vi "test-trajectory-generator-get.vi"(11 "traj_config":T4 {"End Velocity" format="%20.4f"; "StartVelocity" format="%20.4f"; "Max Acceleration" format="%20.4f"; "MaxVelocity" format="%20.4f"}) -> (0 "error out":errorcluster, 3 "TRAJECTORY":T5 {"States"."POSE"."ROTATION"."SIN" format="%13.4f"; "States"."POSE"."ROTATION"."COS" format="%13.4f"; "States"."POSE"."ROTATION"."VALUE" format="%13.4f"; "States"."POSE"."TRANSLATION"."Y" format="%14.3f"; "States"."POSE"."TRANSLATION"."X" format="%14.3f"; "TotalTImeSecs" format="%20.3f"}, 4 "Waypoints":T1[](array[typedef]) {"ROTATION"."SIN" format="%13.4f"; "ROTATION"."COS" format="%13.4f"; "ROTATION"."VALUE" format="%13.4f"; "TRANSLATION"."Y" format="%14.3f"; "TRANSLATION"."X" format="%14.3f"})   [LabVIEW 2019]
uses:
  <vilib>/Rock Robotics/WPI/ThirdParty/JAS_Junk/TrajLib/TRAJECTORY.ctl
  <vilib>/Rock Robotics/WPI/ThirdParty/JAS_Junk/TrajLib/TRAJ_STATE.ctl
  <vilib>/Rock Robotics/WPI/ThirdParty/JAS_Junk/TrajLib/POSE2D.ctl
  <vilib>/Rock Robotics/WPI/ThirdParty/JAS_Junk/TrajLib/TRANSLATION2D.ctl
  <vilib>/Rock Robotics/WPI/ThirdParty/JAS_Junk/TrajLib/ROTATION2D.ctl
  <vilib>/Rock Robotics/WPI/ThirdParty/JAS_Junk/TrajLib/TRAJ_CONFIG.ctl
  <vilib>/Rock Robotics/WPI/ThirdParty/JAS_Junk/TrajLib/DISPLAY_WAYPOINT.ctl
  <vilib>/Rock Robotics/WPI/ThirdParty/JAS_Junk/TrajLib/Rotation2d_CreateAngle.vi
  <vilib>/Rock Robotics/WPI/ThirdParty/JAS_Junk/TrajLib/Pose2d_TransformBy.vi
  <vilib>/Rock Robotics/WPI/ThirdParty/JAS_Junk/TrajLib/Translation2d_RotateBy.vi
  <vilib>/Rock Robotics/WPI/ThirdParty/JAS_Junk/TrajLib/Translation2d_Plus.vi
  <vilib>/Rock Robotics/WPI/ThirdParty/JAS_Junk/TrajLib/Rotation2d_Plus.vi
  <vilib>/Rock Robotics/WPI/ThirdParty/JAS_Junk/TrajLib/Pose2d_New_TRRO.vi
  <vilib>/Rock Robotics/WPI/ThirdParty/JAS_Junk/TrajLib/Rotation2d_RotateBy.vi
  <vilib>/Rock Robotics/WPI/ThirdParty/JAS_Junk/TrajLib/Rotation2d_CreateXY.vi
  <vilib>/Rock Robotics/WPI/ThirdParty/JAS_Junk/TrajLib/Util_CalcDist.vi
  <vilib>/Rock Robotics/WPI/ThirdParty/JAS_Junk/TrajLib/Trajectory_Library.lvlib
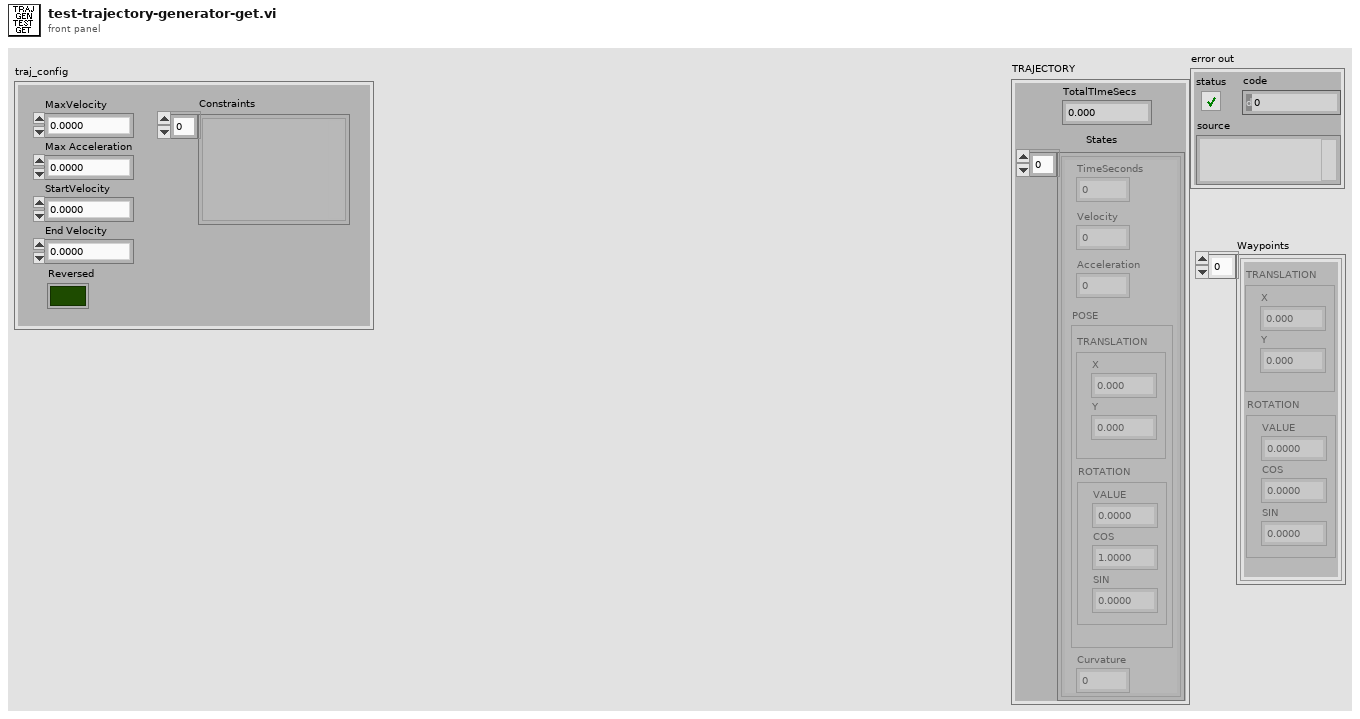
[diagram p1: front panel]
types:
  T1 = typedef "Trajectory_Library.lvlib/POSE2D.ctl" = cluster{"TRANSLATION":T2, "ROTATION":T3}
  T2 = typedef "Trajectory_Library.lvlib/TRANSLATION2D.ctl" = cluster{"X":dbl, "Y":dbl}
  T3 = typedef "Trajectory_Library.lvlib/ROTATION2D.ctl" = cluster{"VALUE":dbl, "COS":dbl, "SIN":dbl}
  T4 = typedef "Trajectory_Library.lvlib/TRAJ_CONFIG.ctl" = cluster{"MaxVelocity":dbl, "Max Acceleration":dbl, "StartVelocity":dbl, "End Velocity":dbl, "Reversed":bool, "Constraints":variant[]}
  T5 = typedef "Trajectory_Library.lvlib/TRAJECTORY.ctl" = cluster{"TotalTImeSecs":dbl, "States":T6[]}
  T6 = typedef "Trajectory_Library.lvlib/TRAJ_STATE.ctl" = cluster{"TimeSeconds":dbl, "Velocity":dbl, "Acceleration":dbl, "POSE":T1, "Curvature":dbl}
  T7 = typedef "Trajectory_Library.lvlib/TRANSFORM2D.ctl" = cluster{"TRANSLATION":T2, "ROTATION":T3, "xF":bool}
  T8 = typedef "Trajectory_Library.lvlib/DISPLAY_WAYPOINT.ctl" = cluster{"X":dbl, "Y":dbl, "ANGLE":dbl}
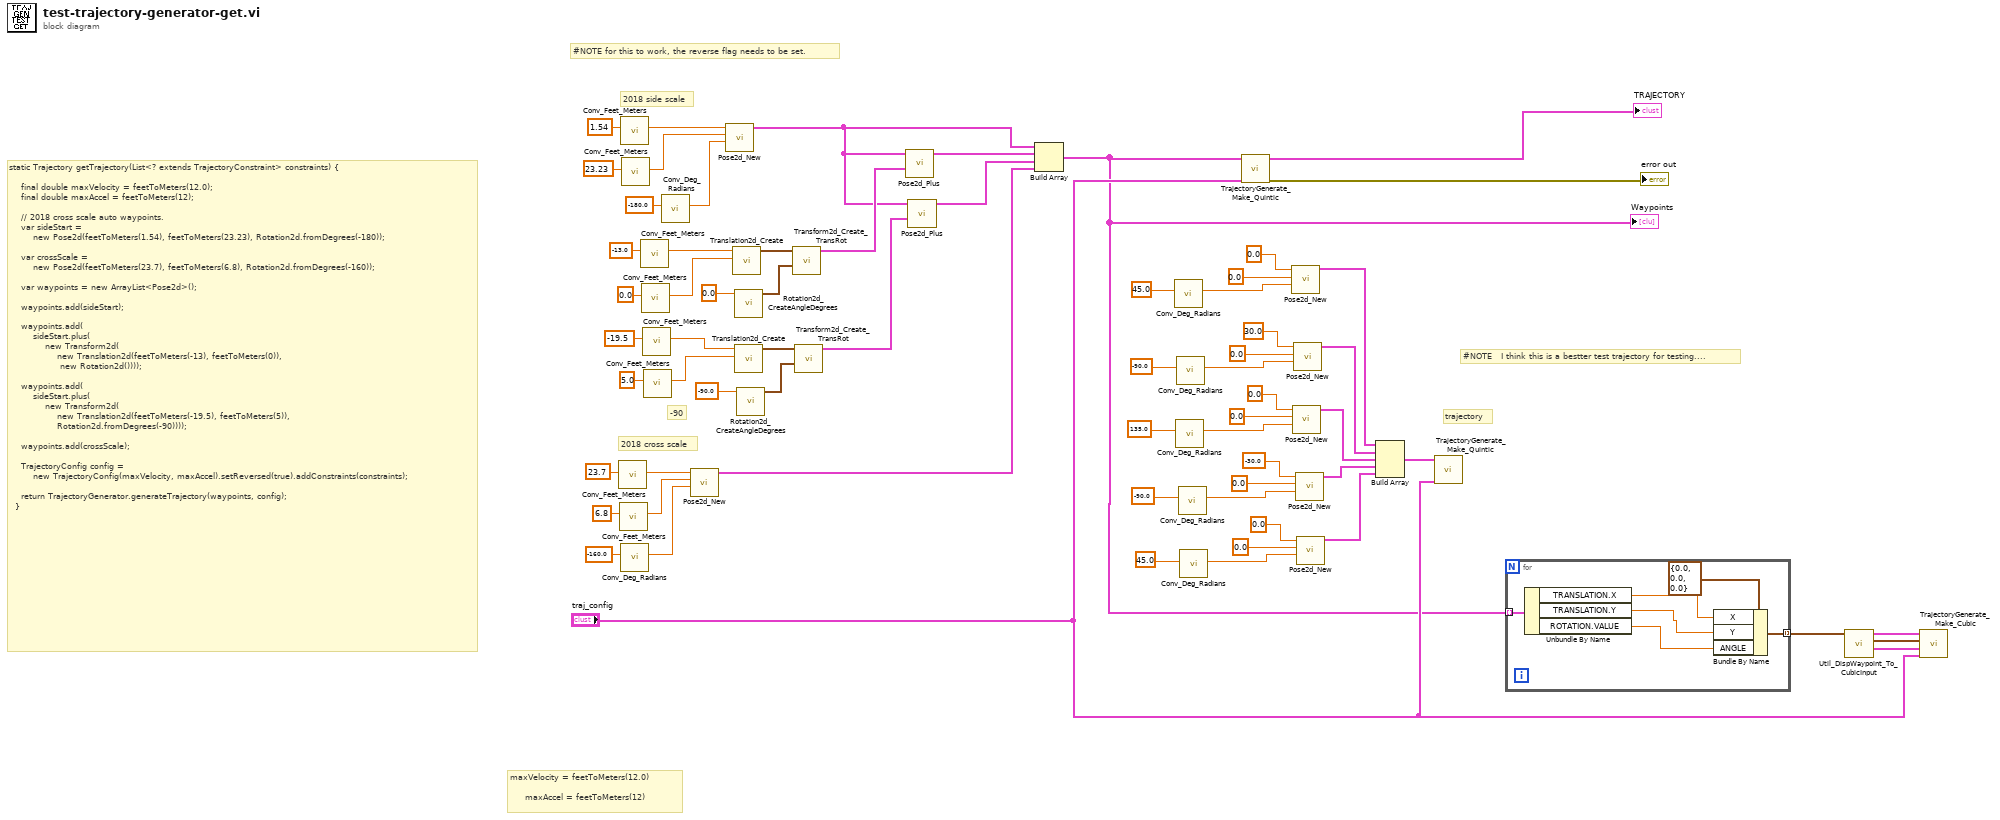
[diagram p0: block diagram]
diagram:
  # "#NOTE for this to work, the reverse flag needs to be set."
  # "-90"
  # "#NOTE   I think this is a bestter test trajectory for testing...."
  # "trajectory"
  # "maxVelocity = feetToMeters(12.0)\n\n     maxAccel = feetToMeters(12)"
  # "2018 cross scale"
  # "2018 side scale"
  # "static Trajectory getTrajectory(List<? extends TrajectoryConstraint> constraints) {\n\n    final double maxVelocity = feetToMeters(12.0);\n    final double maxAccel = feetToMeters(12);\n\n    // 2018 cross scale auto waypoints.\n    var sideStart =\n        new Pose2d(feetToMeters(1.54), feetToMeters(23.23), Rotation2d.fromDegrees(-180));\n\n    var crossScale =\n        new Pose2d(feetToMeters(23.7), feetToMeters(6.8), Rotation2d.fromDegrees(-160));\n\n    var waypoints = new ArrayList<Pose2d>();\n\n    waypoints.add(sideStart);\n\n    waypoints.add(\n        sideStart.plus(\n            new Transform2d(\n                new Translation2d(feetToMeters(-13), feetToMeters(0)), \n                 new Rotation2d())));\n\n    waypoints.add(\n        sideStart.plus(\n            new Transform2d(\n                new Translation2d(feetToMeters(-19.5), feetToMeters(5)),\n                Rotation2d.fromDegrees(-90))));\n\n    waypoints.add(crossScale);\n\n    TrajectoryConfig config =\n        new TrajectoryConfig(maxVelocity, maxAccel).setReversed(true).addConstraints(constraints);\n\n    return TrajectoryGenerator.generateTrajectory(waypoints, config);\n  }"
  n1 = call <vilib>:"Conv_Feet_Meters.vi"("Feet"=23.7) -> ("Meters"=w60:dbl)  [unwired: 10 in]
  n2 = call <vilib>:"Conv_Feet_Meters.vi"("Feet"=6.8) -> ("Meters"=w59:dbl)  [unwired: 10 in]
  n3 = call <vilib>:"Conv_Feet_Meters.vi"("Feet"=1.54) -> ("Meters"=w66:dbl)  [unwired: 10 in]
  n4 = call <vilib>:"Conv_Deg_Radians.vi"("Degress"=-160.0) -> ("Radians"=w58:dbl)  [unwired: 10 in]
  n5 = call <vilib>:"Conv_Feet_Meters.vi"("Feet"=23.23) -> ("Meters"=w65:dbl)  [unwired: 10 in]
  n6 = call <vilib>:"Conv_Feet_Meters.vi"("Feet"=-13.0) -> ("Meters"=w38:dbl)  [unwired: 10 in]
  n7 = call <vilib>:"Conv_Feet_Meters.vi"("Feet"=0.0) -> ("Meters"=w37:dbl)  [unwired: 10 in]
  n8 = call <vilib>:"Conv_Feet_Meters.vi"("Feet"=-19.5) -> ("Meters"=w36:dbl)  [unwired: 10 in]
  n9 = call <vilib>:"Conv_Feet_Meters.vi"("Feet"=5.0) -> ("Meters"=w35:dbl)  [unwired: 10 in]
  n10 = call <vilib>:"Conv_Deg_Radians.vi"("Degress"=-180.0) -> ("Radians"=w64:dbl)  [unwired: 10 in]
  n11 = call <vilib>:"Pose2d_New.vi"("Heading"=w58, "Y"=w59, "X"=w60) -> ("out POSe"=w54:T1)  [unwired: 8 in]
  n12 = call <vilib>:"Pose2d_New.vi"("Heading"=w64, "Y"=w65, "X"=w66) -> ("out POSe"=w45:T1)  [unwired: 8 in]
  n13 = call <vilib>:"Translation2d_Create.vi"("Y"=w37, "X"=w38) -> ("TRANSLATION"=w53:T2)  [unwired: 9 in]
  n14 = call <vilib>:"Rotation2d_CreateAngleDegrees.vi"("Angle_Degrees"=0.0) -> ("ROTATION"=w52:T3)  [unwired: 10 in]
  n15 = call <vilib>:"Translation2d_Create.vi"("Y"=w35, "X"=w36) -> ("TRANSLATION"=w48:T2)  [unwired: 9 in]
  n16 = call <vilib>:"Rotation2d_CreateAngleDegrees.vi"("Angle_Degrees"=-90.0) -> ("ROTATION"=w47:T3)  [unwired: 10 in]
  n17 = call <vilib>:"Transform2d_Create_TransRot.vi"("ROTATION"=w52, "TRANSLATION"=w53) -> ("TRANSFORM"=w50:T7)  [unwired: 9 in]
  n18 = call <vilib>:"Transform2d_Create_TransRot.vi"("ROTATION"=w47, "TRANSLATION"=w48) -> ("TRANSFORM"=w44:T7)  [unwired: 9 in]
  n19 = call <vilib>:"Pose2d_Plus.vi"("other TRANSFORM"=w50, "in POSE"=w45) -> ("out POSE"=w49:T1)  [unwired: 9 in]
  n20 = call <vilib>:"Pose2d_Plus.vi"("other TRANSFORM"=w44, "in POSE"=w45) -> ("out POSE"=w43:T1)  [unwired: 9 in]
  n21 = Build Array(w45, w49, w43, w54) -> (w3:T1[])
  "Waypoints" <- w3
  n22 = call <vilib>:"Conv_Deg_Radians.vi"("Degress"=45.0 ("Heading")) -> ("Radians"=w10:dbl)  [unwired: 10 in]
  n23 = call <vilib>:"Conv_Deg_Radians.vi"("Degress"=135.0 ("Heading")) -> ("Radians"=w18:dbl)  [unwired: 10 in]
  n24 = call <vilib>:"Conv_Deg_Radians.vi"("Degress"=-90.0 ("Heading")) -> ("Radians"=w14:dbl)  [unwired: 10 in]
  n25 = call <vilib>:"Conv_Deg_Radians.vi"("Degress"=-90.0 ("Heading")) -> ("Radians"=w22:dbl)  [unwired: 10 in]
  n26 = call <vilib>:"Conv_Deg_Radians.vi"("Degress"=45.0 ("Heading")) -> ("Radians"=w26:dbl)  [unwired: 10 in]
  n27 = call <vilib>:"TrajectoryGenerate_Make_Quintic.vi"("traj_config"="traj_config", "waypointPOSE"=w3) -> ("error out"=→"error out":errorcluster, "TRAJECTORY"=→"TRAJECTORY":T5)  [unwired: 8 in]
  n28 = call <vilib>:"Pose2d_New.vi"("Heading"=w10, "Y"=0.0, "X"=0.0) -> ("out POSe"=w9:T1)  [unwired: 8 in]
  n29 = call <vilib>:"Pose2d_New.vi"("Heading"=w18, "Y"=0.0, "X"=0.0) -> ("out POSe"=w7:T1)  [unwired: 8 in]
  n30 = call <vilib>:"Pose2d_New.vi"("Heading"=w14, "Y"=0.0, "X"=30.0) -> ("out POSe"=w8:T1)  [unwired: 8 in]
  n31 = call <vilib>:"Pose2d_New.vi"("Heading"=w22, "Y"=0.0, "X"=-30.0) -> ("out POSe"=w6:T1)  [unwired: 8 in]
  n32 = call <vilib>:"Pose2d_New.vi"("Heading"=w26, "Y"=0.0, "X"=0.0) -> ("out POSe"=w28:T1)  [unwired: 8 in]
  n33 = Build Array(w9, w8, w7, w6, w28) -> (w4:T1[])
  n34 = call <vilib>:"TrajectoryGenerate_Make_Quintic.vi"("traj_config"="traj_config", "waypointPOSE"=w4) -> ()  [unwired: 8 in, 2 out]
  n35 = for {
    tunnel: w3 -> [w72] mode=indexing
    tunnel: [w67] -> w31 mode=indexing
    n36 = Unbundle By Name(w72) -> ("TRANSLATION.X"=w68:dbl, "TRANSLATION.Y"=w69:dbl, "ROTATION.VALUE"=w70:dbl)
    n37 = Bundle By Name(cluster=T8 {"X"=0.0, "Y"=0.0, "ANGLE"=0.0} ("UTIL_WAYPOINT"), "X"=w68, "Y"=w69, "ANGLE"=w70) -> (w67:T8)
  }
  n38 = call <vilib>:"Util_DispWaypoint_To_CubicInput.vi"("WayPoints"=w31) -> ("Final POSE"=w32:T1, "Internal Cubic Waypoints"=w33:T2[], "Initial POSE"=w34:T1)  [unwired: 8 in]
  n39 = call <vilib>:"TrajectoryGenerate_Make_Cubic.vi"("traj_config"="traj_config", "Enging POSE"=w32, "Interior WAYPOINTS"=w33, "Starting POSE"=w34) -> ()  [unwired: 6 in, 2 out]
